vi "calibration.vi"() -> ()   [LabVIEW 2013]
uses:
  <vilib>/Analysis/polynomials.llb/Scalar Polynomial Evaluation (DBL).vi
  <vilib>/Analysis/NI_AALPro.lvlib
panel:
  out "x+y":sgl
  out "Polynomial Coefficients":dbl[](array[numeric])
  out "P(a)":dbl
  in  "a":sgl
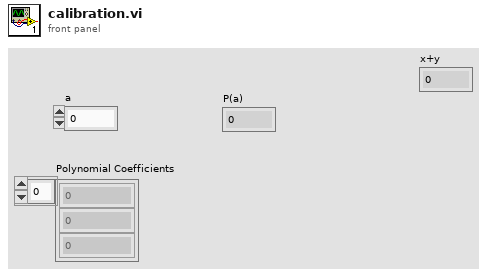
[diagram p1: front panel]
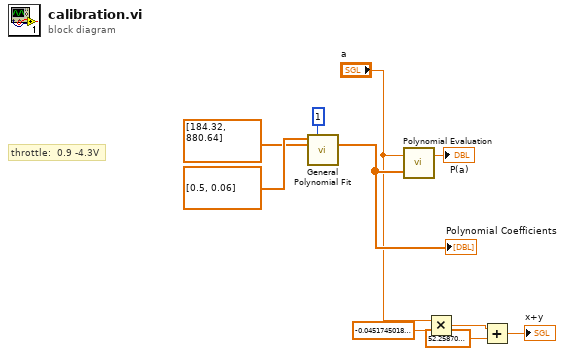
[diagram p0: block diagram]
diagram:
  # "throttle:  0.9 -4.3V"
  n1 = call <vilib>:"General Polynomial Fit.vi"("Y"=dbl[] [0.5, 0.06], "polynomial order"=1, "X"=dbl[] [184.32, 880.64] ("Y")) -> ("Polynomial Coefficients"=w6:dbl[])  [unwired: 9 in, 3 out]
  "Polynomial Coefficients" <- w6
  n2 = call-poly <vilib>:"Polynomial Evaluation.vi"("P(x)"=w6, "a"="a") -> ("P(a)"=→"P(a)":dbl)  [unwired: 1 out]
  n3 = Multiply(x="a", y=sgl -0.0451745) -> (x*y=w4:sgl)
  n4 = Add(x=w4, y=sgl 52.2587) -> (x+y=→"x+y":sgl)
